vi "Write Label Names.vi"(8 "error in (no error)":errorcluster, 10 "Label Names":string[](array[string]), 11 "Metric in":refnum<class "Metric.lvclass">) -> (0 "error out":errorcluster, 3 "Metric out":refnum<class "Metric.lvclass">)   [LabVIEW 2020, in "Metrics.lvlib" / "Metric.lvclass"]
uses:
  Metric.lvclass
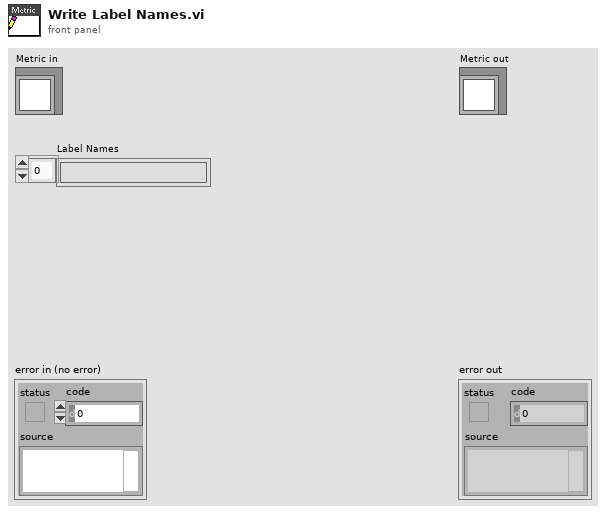
[diagram p1: front panel]
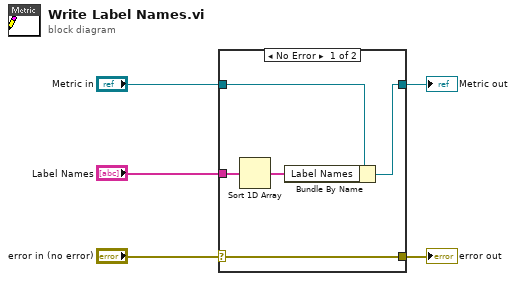
[diagram p0: block diagram]
diagram:
  n1 = case shown="No Error" "error in (no error)" {
    selector: "error in (no error)" -> [w10 w11]
    tunnel: [w10 w11] -> w4
    tunnel: [w8 w12] -> w2
    tunnel: "Metric in" -> [w9 w12]
    tunnel: "Label Names" -> [w7 _]
    frame No Error {
      n2 = Sort 1D Array(array=w7) -> (sorted array=w6:string[])
      n3 = Bundle By Name(cluster=w9, "Label Names"=w6) -> (w8:refnum<class "Metric.lvclass">)
    }
    frame Error {
    }
  }
  "error out" <- w4
  "Metric out" <- w2
